vi "Loader Animation.vi"(0 "vi reference":refnum<vi>, 11 "error in (no error)":errorcluster, 12 "animation on":bool=TRUE) -> (15 "error out":errorcluster)   [LabVIEW 2016]
doc: "Shows and hides front panel specifed on a <b>vi reference</b>, in a special method.\n\n\n------------------------------\nPawe³ Pawlik 26.01.2010\npawlik.pawel@gmail.com"
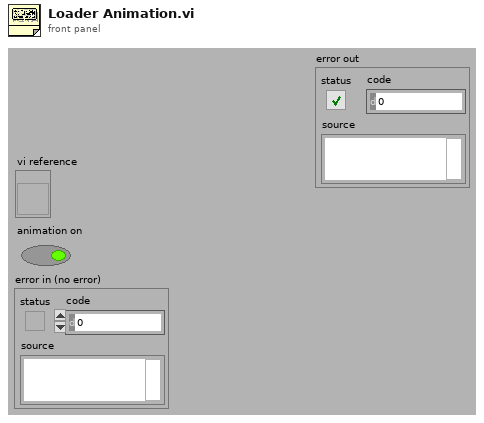
[diagram p1: front panel]
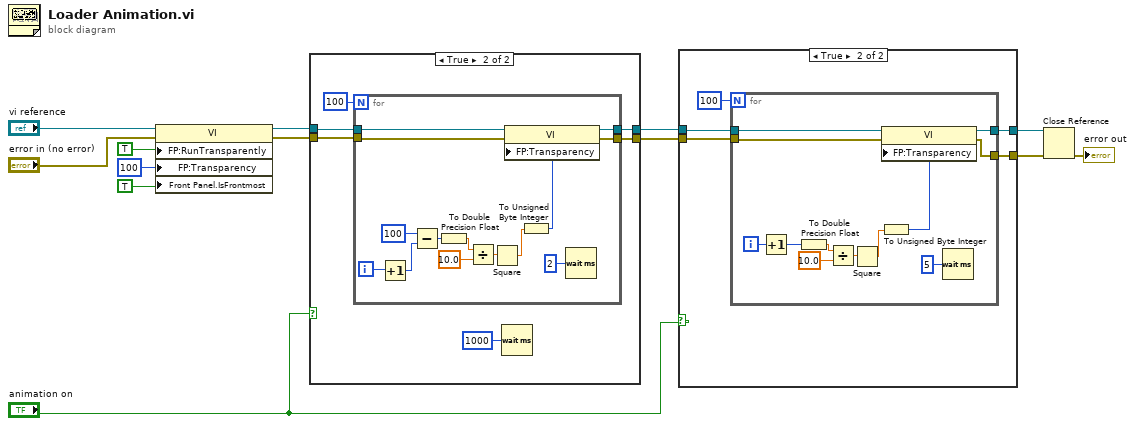
[diagram p0: block diagram]
diagram:
  n1 = property class="VI"(reference="vi reference", error in="error in (no error)", "FP:RunTransparently"=TRUE ("Front Panel Window:Run VI Transparently"), "FP:Transparency"=u8 100 ("Front Panel Window:Transparency"), "Front Panel.IsFrontmost"=TRUE ("Front Panel Window:Is Frontmost")) -> (reference out=w11:refnum<vi>, error out=w10:errorcluster)
  n2 = case shown="True" "animation on" {
    tunnel: w11 -> [w15 w20]
    tunnel: [w15 w19] -> w6
    tunnel: [w14 w18] -> w5
    tunnel: w10 -> [w14 w17]
    frame False {
    }
    frame True {
      n3 = for {
        N: 100 -> [_]
        tunnel: [w35] -> w19
        tunnel: w20 -> [w34]
        tunnel: w17 -> [w32]
        tunnel: [w29] -> w18
        i -> [w22]
        n4 = Increment(x=w22) -> (x+1=w23:i32)
        n5 = Subtract(x=100, y=w23) -> (x-y=w26:i32)
        n6 = To Double Precision Float(number=w26) -> (double precision float=w27:dbl)
        n7 = Divide(x=w27, y=10.0) -> (x/y=w30:dbl)
        n8 = Square(x=w30) -> (x^2=w25:dbl)
        n9 = To Unsigned Byte Integer(number=w25) -> (unsigned 8bit integer=w24:u8)
        n10 = property class="VI"(reference=w34, error in=w32, "FP:Transparency"=w24) -> (reference out=w35:refnum<vi>, error out=w29:errorcluster)
        n11 = Wait (ms)(milliseconds to wait=u32 2) -> ()  [unwired: 1 out]
      }
      n12 = Wait (ms)(milliseconds to wait=u32 1000 ("millisecond multiple")) -> ()  [unwired: 1 out]
    }
  }
  n13 = case shown="True" "animation on" {
    tunnel: w6 -> [w37 w41]
    tunnel: [w37 w40] -> w3
    tunnel: [w36 w39] -> w2
    tunnel: w5 -> [w36 w38]
    frame False {
    }
    frame True {
      n14 = for {
        N: 100 -> [_]
        tunnel: [w54] -> w40
        tunnel: w41 -> [w53]
        tunnel: w38 -> [w51]
        tunnel: [w48] -> w39
        i -> [w43]
        n15 = Increment(x=w43) -> (x+1=w44:i32)
        n16 = To Double Precision Float(number=w44) -> (double precision float=w47:dbl)
        n17 = Divide(x=w47, y=10.0) -> (x/y=w49:dbl)
        n18 = Square(x=w49) -> (x^2=w46:dbl)
        n19 = To Unsigned Byte Integer(number=w46) -> (unsigned 8bit integer=w45:u8)
        n20 = property class="VI"(reference=w53, error in=w51, "FP:Transparency"=w45) -> (reference out=w54:refnum<vi>, error out=w48:errorcluster)
        n21 = Wait (ms)(milliseconds to wait=u32 5) -> ()  [unwired: 1 out]
      }
    }
  }
  n22 = Close Reference(reference=w3, error in (no error)=w2) -> (error out=→"error out":errorcluster)
